vi "T_kulso_levego.vi"(6 "mód":enum16{"szinusz", "ugrás"}(ring), 8 "T_min":dbl=20.5, 9 "T_max":dbl=33.5, 10 "t_vektor":dbl[](array[numeric])) -> (1 "T_atlag":dbl format="%0.2f", 2 "T_kulso_levego_vektor":dbl[](array[numeric]))   [LabVIEW 2013]
uses:
  <vilib>/Analysis/baseanly.llb/Mean (DBL).vi
  <vilib>/Analysis/NI_AALBase.lvlib
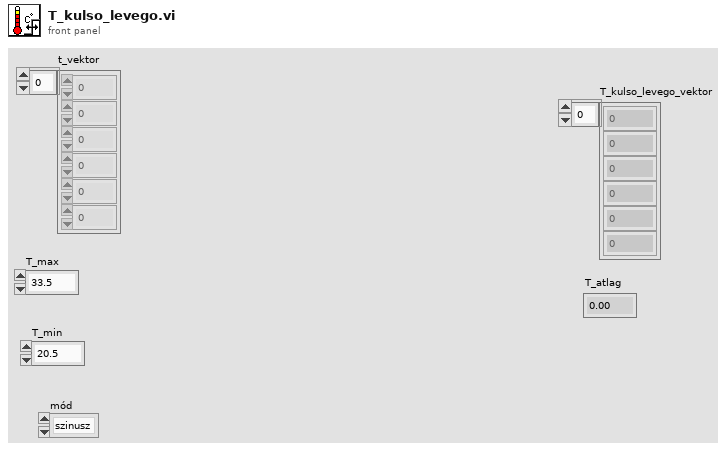
[diagram p1: front panel]
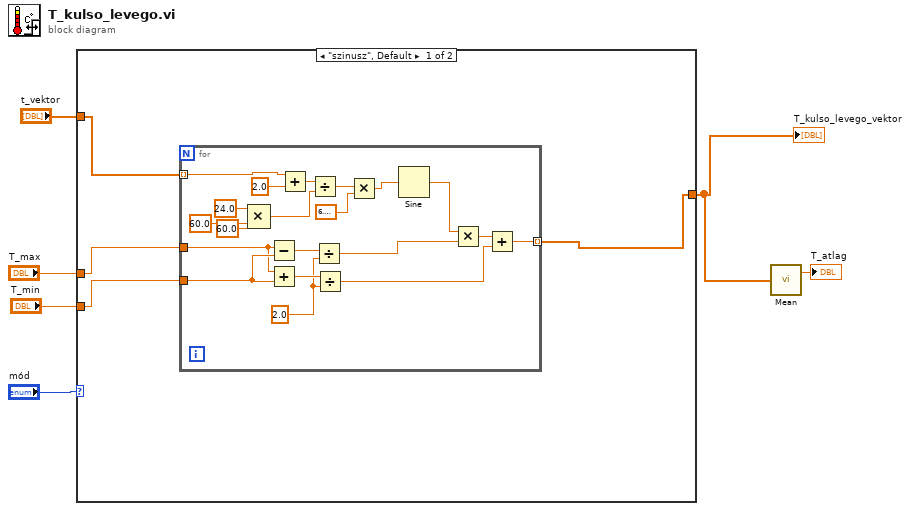
[diagram p0: block diagram]
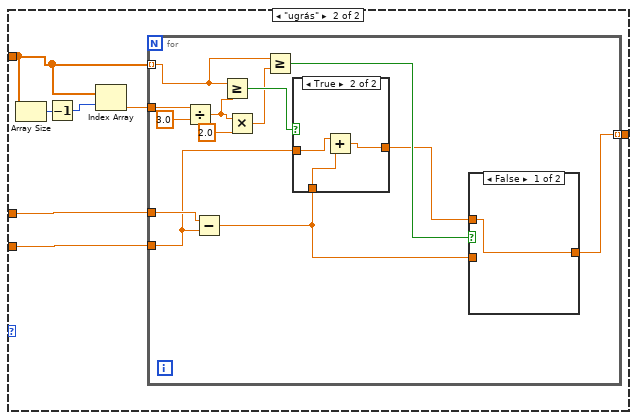
[diagram p2: hidden frame]
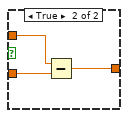
[diagram p3: hidden frame]
diagram:
  n1 = case shown="\"szinusz\", Default" "mód" {
    tunnel: "T_max" -> [w8 w37]
    tunnel: "T_min" -> [w7 w36]
    tunnel: [w9 w35] -> w4
    tunnel: "t_vektor" -> [w10 w34]
    frame "szinusz", Default {
      n2 = for {
        tunnel: w10 -> [w22] mode=indexing
        tunnel: w8 -> [w29]
        tunnel: w7 -> [w30]
        tunnel: [w18] -> w9 mode=indexing
        w26 = 2.0
        n3 = Compound Arithmetic op=MULTIPLY(24.0, 60.0 ("value"), 60.0 ("value")) -> (w11:dbl)
        n4 = Subtract(x=w29, y=w30) -> (x-y=w28:dbl)
        n5 = Add(x=w29, y=w30) -> (x+y=w27:dbl)
        n6 = Add(x=w22, y=2.0) -> (x+y=w21:dbl)
        n7 = Divide(x=w21, y=w11) -> (x/y=w17:dbl)
        n8 = Divide(x=w28, y=w26) -> (x/y=w24:dbl)
        n9 = Divide(x=w27, y=w26) -> (x/y=w19:dbl)
        n10 = Multiply(x=w17, y=6.283185307179586) -> (x*y=w16:dbl)
        n11 = Sine(x=w16) -> (sin(x)=w25:dbl)
        n12 = Multiply(x=w25, y=w24) -> (x*y=w20:dbl)
        n13 = Add(x=w20, y=w19) -> (x+y=w18:dbl)
      }
    }
    frame "ugrás" {
      n14 = Array Size(array=w34) -> (size(s)=w33:i32)
      n15 = Decrement(x=w33) -> (x-1=w32:i32)
      n16 = Index Array(array=w34, index=w32) -> (element=w31:dbl)
      n17 = for {
        tunnel: w34 -> [w42] mode=indexing
        tunnel: w37 -> [w47]
        tunnel: w36 -> [w46]
        tunnel: [w39] -> w35 mode=indexing
        tunnel: w31 -> [w50]
        n18 = Divide(x=w50, y=3.0) -> (x/y=w45:dbl)
        n19 = Subtract(x=w47, y=w46) -> (x-y=w38:dbl)
        n20 = Greater Or Equal?(x=w42, y=w45) -> (x >= y?=w48:bool)
        n21 = Multiply(x=w45, y=2.0) -> (x*y=w43:dbl)
        n22 = Greater Or Equal?(x=w42, y=w43) -> (x >= y?=w41:bool)
        n23 = case shown="True" w48 {
          tunnel: w46 -> [w55 w58]
          tunnel: w38 -> [_ w57]
          tunnel: [w55 w56] -> w40
          frame False {
          }
          frame True {
            n24 = Add(x=w58, y=w57) -> (x+y=w56:dbl)
          }
        }
        n25 = case shown="False" w41 {
          tunnel: w40 -> [w51 w54]
          tunnel: [w51 w53] -> w39
          tunnel: w38 -> [_ w52]
          frame False {
          }
          frame True {
            n26 = Subtract(x=w54, y=w52) -> (x-y=w53:dbl)
          }
        }
      }
    }
  }
  "T_kulso_levego_vektor" <- w4
  n27 = call-poly <vilib>:"Mean.vi"("X"=w4) -> ("mean"=→"T_atlag":dbl)  [unwired: 1 out]
